vi "Display Two Button Popup.vi"(5 "N-Text":string="No", 6 "Theme":refnum<class "Theme.lvclass">, 7 "Y-Text":string="Yes", 8 "error in":errorcluster, 10 "Message":string, 11 "Graphic":T1="info") -> (0 "error out":errorcluster, 1 "Choice":bool)   [LabVIEW 2021, in "Pop-Up.lvlib" / "Two Button.lvclass"]
doc: "The two button popup will display information to the user and wait for the operator to choose a button.\n\n<b>Note:</b> The function <b>Close Pop-Up (Two Button Choice).vi</b> can be used to close this dialog early and send a value for the choice of Boolean selection. Otherwise, to just close the dialog early, use Close Pop-Up.vi.\n\nInputs:\n-Graphic [typedef combobox] - Image (PNG) for Graphic for Popup\n-Message [String] - String Variable to populate Display\n-Theme [lvclass] - the theme for the style of the popup\n-YText [string] - the string for the YES button\n-NText [string] - the string for the NO button\n\nOutputs\n-Choice [boolean] - the option that was chosen by the user\n\n<b>Code Developed By:</b>\nDaniel Coons\nTechnology Service Corporation\n1983 S Liberty Drive\nBloomington, IN 47403\nPhone: 812 558-7100\ndaniel.coons@tsc.com\nwww.tsc.com/atcs"
uses:
  Two Button.lvclass
  Theme/Theme.lvclass
  Graphics.ctl
  C:/Development/Open Source/tsc-pop-up/Popup/Popup.lvclass
  Two Button.lvclass/Two Button.ctl
  Pop-Up.lvlib
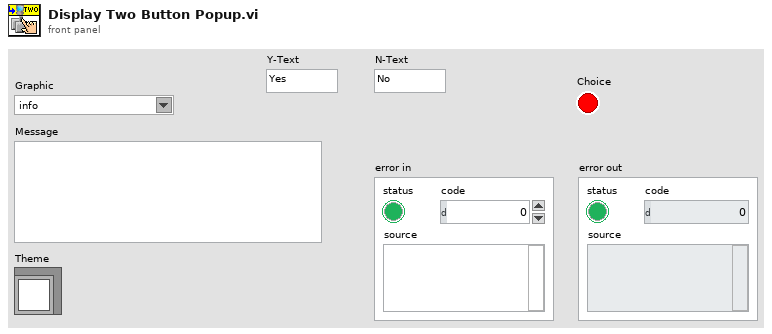
[diagram p1: front panel]
types:
  T1 = typedef "Pop-Up.lvlib/Graphics.ctl" = string
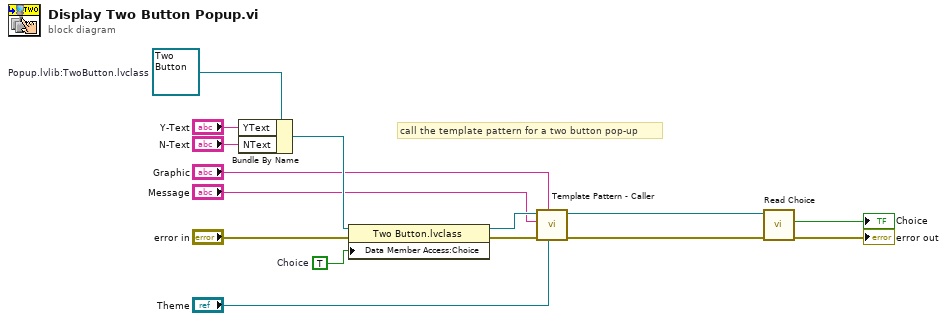
[diagram p0: block diagram]
diagram:
  w5 = TRUE  # Choice
  w10 = refnum<class "Two Button.lvclass"> refnum  # Popup.lvlib:TwoButton.lvclass
  # "call the template pattern for a two button pop-up"
  n1 = Bundle By Name(cluster=w10, "YText"="Y-Text", "NText"="N-Text") -> (w7:refnum<class "Two Button.lvclass">)
  n2 = property class="Two Button.lvclass"(reference=w7, error in="error in", "Data Member Access:Choice"=w5) -> (reference out=w6:refnum<class "Two Button.lvclass">, error out=w8:errorcluster)
  n3 = call-dynamic "Template Pattern - Caller.vi"("Theme"="Theme", "standard"="Graphic", "error in (no error)"=w8, "Message"="Message", "Pop-Up in"=w6) -> ("error out"=w11:errorcluster, "Pop-Up out"=w1:refnum<class "Two Button.lvclass">)  [unwired: 5 in]
  n4 = call-dynamic "Read Choice.vi"("error in (no error)"=w11, "_Popup in"=w1) -> ("error out"=→"error out":errorcluster, "Choice"=→"Choice":bool)  [unwired: 7 in, 1 out]
